vi "Not A Session.vi"(1 "session":T1) -> (0 "Not a Session?":bool)   [LabVIEW 2013, in "libssh2.lvlib"]
doc: "Returns TRUE if <B>session</B> is not a session. Otherwise, this function returns FALSE."
uses:
  libssh2.lvlib
  Session Refnum.ctl
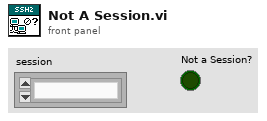
[diagram p1: front panel]
types:
  T1 = typedef "libssh2.lvlib/Session Refnum.ctl" = refnum<k1>
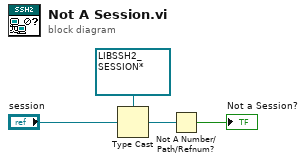
[diagram p0: block diagram]
diagram:
  n1 = Type Cast(type=refnum<data-value> refnum ("data value reference"), x="session") -> (*(type *) &x=w2:refnum<data-value>)
  n2 = Not A Number/Path/Refnum?(number/path/refnum=w2) -> (NaN/Path/Refnum?=→"Not a Session?":bool)
